vi "9_Calculate output_solution.vi"(11 "Input":u32) -> (3 "Output":u32)   [LabVIEW 2014]
panel:
  # "calculate the output according to the example\nthe input will be no more than 100000"
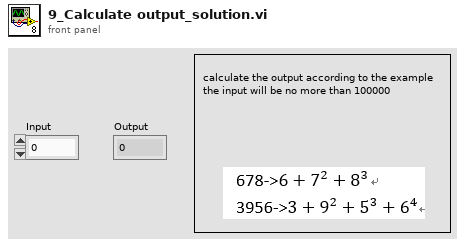
[diagram p1: front panel]
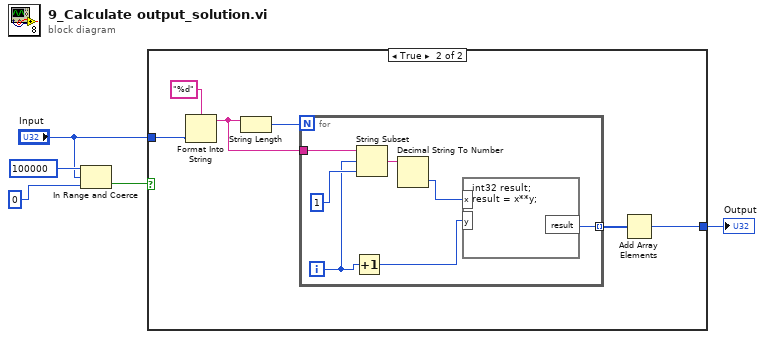
[diagram p0: block diagram]
diagram:
  n1 = In Range and Coerce(upper limit=100000, x="Input", lower limit=0) -> (In Range?=w3:bool)  [unwired: 1 out]
  n2 = case shown="True" w3 {
    tunnel: "Input" -> [_ w11]
    tunnel: [_ w6] -> w1
    frame False {
    }
    frame True {
      n3 = Format Into String(format string="%d", w11) -> (resulting string=w8:string)  [unwired: 2 in, 1 out]
      n4 = String Length(string=w8) -> (length=w9:i32)
      n5 = for {
        N: w9 -> [_]
        tunnel: w8 -> [w18]
        tunnel: [w12] -> w7 mode=indexing
        i -> [w15]
        n6 = Increment(x=w15) -> (x+1=w14:i32)
        n7 = String Subset(string=w18, offset (0)=w15, length (rest)=1) -> (substring=w17:string)
        n8 = Decimal String To Number(string=w17) -> (number=w13:i32)  [unwired: 2 in, 1 out]
        n9 = formula code="int32 result;\nresult = x**y;"("x"=w13, "y"=w14) -> ("result"=w12:i32)
      }
      n10 = Add Array Elements(numeric array=w7) -> (sum=w6:i32)
    }
  }
  "Output" <- w1
